vi "Import.vi"(8 "error in":errorcluster, 10 "path":path, 11 "item to replace":T1 format="%.0x") -> (0 "error out":errorcluster, 3 "new item":T1 format="%.0x")   [LabVIEW 2017, in "Import Export.lvlib"]
uses:
  Import Export.lvlib
  <vilib>/NI Veristand/Custom Device API/Custom Device Item Ref.ctl
  System Explorer Action.ctl
  NationalInstruments.VeriStand.SystemDefinitionAPI
  NationalInstruments.VeriStand.SystemStorage
  <vilib>/NI Veristand/Custom Device API/Custom Device API.lvlib
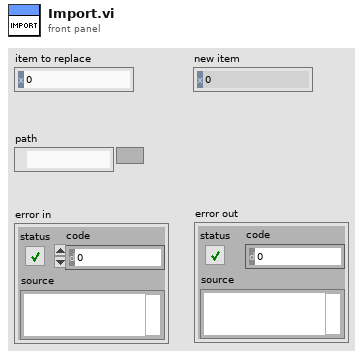
[diagram p1: front panel]
types:
  T1 = typedef "Custom Device API.lvlib/Custom Device Item Ref.ctl" = u64
  T2 = typedef "Import Export.lvlib/System Explorer Action.ctl" = u16
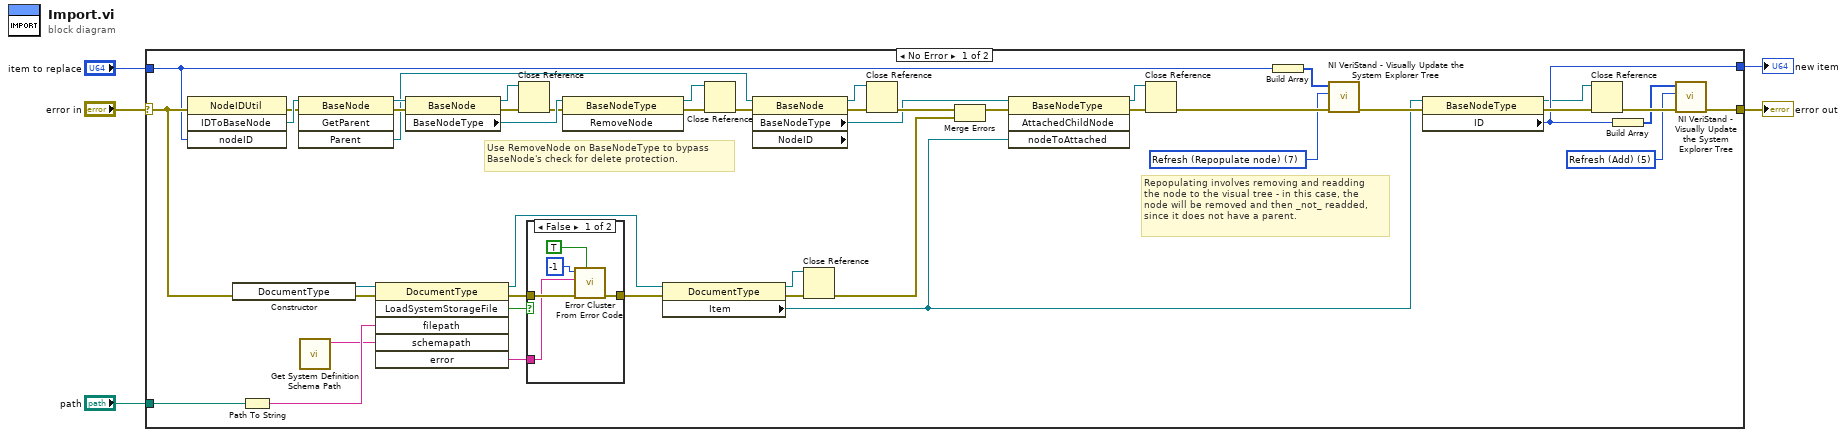
[diagram p0: block diagram]
diagram:
  n1 = case shown="No Error" "error in" {
    selector: "error in" -> [w29 w58]
    tunnel: "path" -> [w46 _]
    tunnel: [w14 w58] -> w3
    tunnel: "item to replace" -> [w13 _]
    tunnel: [w8 _] -> w1
    frame No Error {
      w9 = T2 7 items=["Refresh (Add)"=5, "Refresh (Repopulate node)"=7, "Refresh (Delete)"=9] ("Action")
      w10 = T2 5 items=["Refresh (Add)"=5, "Refresh (Repopulate node)"=7, "Refresh (Delete)"=9] ("Action")
      # "Repopulating involves removing and readding\nthe node to the visual tree - in this case, the\nnode will be removed and then _not_ readded,\nsince it does not have a parent."
      # "Use RemoveNode on BaseNodeType to bypass\nBaseNode's check for delete protection."
      n2 = invoke class="NodeIDUtil" method="IDToBaseNode"(error in=w29, "nodeID"=w13) -> (error out=w39:errorcluster, "IDToBaseNode"=w41:refnum<k24>)  [unwired: 2 in, 2 out]
      n3 = constructor class="DocumentType"(error in=w29) -> (reference out=w24:refnum<k24>, error out=w25:errorcluster)  [unwired: 2 in, 1 out]
      n4 = Path To String(path=w46) -> (string=w23:string)
      n5 = invoke class="BaseNode" method="GetParent"(reference=w41, error in=w39) -> (reference out=w38:refnum<k24>, error out=w40:errorcluster, "Parent"=w37:refnum<k24>)  [unwired: 2 in, 1 out]
      n6 = call "Get System Definition Schema Path.vi"() -> ("system definition schema path"=w22:string)  [unwired: 11 in]
      n7 = invoke class="DocumentType" method="LoadSystemStorageFile"(reference=w24, error in=w25, "filepath"=w23, "schemapath"=w22) -> (reference out=w17:refnum<k24>, error out=w21:errorcluster, "LoadSystemStorageFile"=w18:bool, "error"=w19:string)  [unwired: 2 in, 2 out]
      n8 = property class="BaseNode"(reference=w38, error in=w40) -> (reference out=w35:refnum<k24>, error out=w44:errorcluster, "BaseNodeType"=w42:refnum<k24>)
      n9 = Close Reference(reference=w35, error in (no error)=w44) -> (error out=w36:errorcluster)
      n10 = case shown="False" w18 {
        tunnel: [w54 w57] -> w20
        tunnel: w21 -> [w55 w57]
        tunnel: w19 -> [w52 _]
        frame False {
          n11 = call <vilib>:"Error Cluster From Error Code.vi"("show call chain? (False)"=TRUE, "error in (no error)"=w55, "error message (\"\")"=w52, "error code (0)"=-1) -> ("error out"=w54:errorcluster)  [unwired: 5 in]
        }
        frame True {
        }
      }
      n12 = invoke class="BaseNodeType" method="RemoveNode"(reference=w42, error in=w36) -> (reference out=w33:refnum<k24>, error out=w45:errorcluster)  [unwired: 1 in, 1 out]
      n13 = property class="DocumentType"(reference=w17, error in=w20) -> (reference out=w26:refnum<k24>, error out=w31:errorcluster, "Item"=w15:refnum<k24>)
      n14 = Close Reference(reference=w33, error in (no error)=w45) -> (error out=w34:errorcluster)
      n15 = property class="BaseNode" props=["BaseNodeType", "NodeID"](reference=w37, error in=w34) -> (reference out=w28:refnum<k24>, error out=w32:errorcluster, "BaseNodeType"=w43:refnum<k24>)  [unwired: 1 out]
      n16 = Close Reference(reference=w26, error in (no error)=w31) -> (error out=w27:errorcluster)
      n17 = Close Reference(reference=w28, error in (no error)=w32) -> (error out=w51:errorcluster)
      n18 = Merge Errors(w51, w27) -> (w30:errorcluster)
      n19 = invoke class="BaseNodeType" method="AttachedChildNode"(reference=w43, error in=w30, "nodeToAttached"=w15) -> (reference out=w16:refnum<k24>, error out=w7:errorcluster)  [unwired: 1 in, 2 out]
      n20 = Close Reference(reference=w16, error in (no error)=w7) -> (error out=w50:errorcluster)
      n21 = Build Array(w13) -> (w12:T1[])
      n22 = call "NI VeriStand - Visually Update the System Explorer Tree.vi"("error in (no error)"=w50, "Action"=w9, "Node IDs"=w12) -> ("error out"=w49:errorcluster)  [unwired: 8 in]
      n23 = property class="BaseNodeType"(reference=w15, error in=w49) -> (reference out=w6:refnum<k24>, error out=w48:errorcluster, "ID"=w8:u64)
      n24 = Close Reference(reference=w6, error in (no error)=w48) -> (error out=w47:errorcluster)
      n25 = Build Array(w8) -> (w11:u64[])
      n26 = call "NI VeriStand - Visually Update the System Explorer Tree.vi"("error in (no error)"=w47, "Action"=w10, "Node IDs"=w11) -> ("error out"=w14:errorcluster)  [unwired: 8 in]
    }
    frame Error {
    }
  }
  "error out" <- w3
  "new item" <- w1
